vi "COMMAND_GetError.vi"(8 "error in (no error)":errorcluster, 11 "StageMH100301DMC in":refnum<class "StageMH100301DMC.lvclass">) -> (0 "error out":errorcluster, 3 "StageMH100301DMC out":refnum<class "StageMH100301DMC.lvclass">)   [LabVIEW 2010, in "StageMH100301DMC.lvclass"]
uses:
  StageMH100301DMC.lvclass
  StageMH100301DMC.lvclass/StageMH100301DMC.ctl
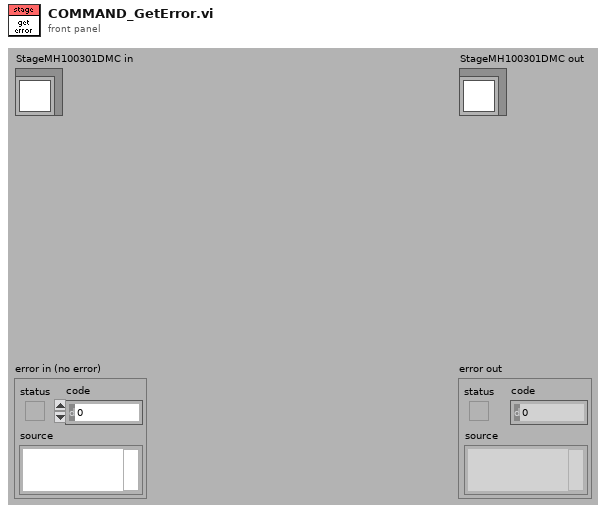
[diagram p1: front panel]
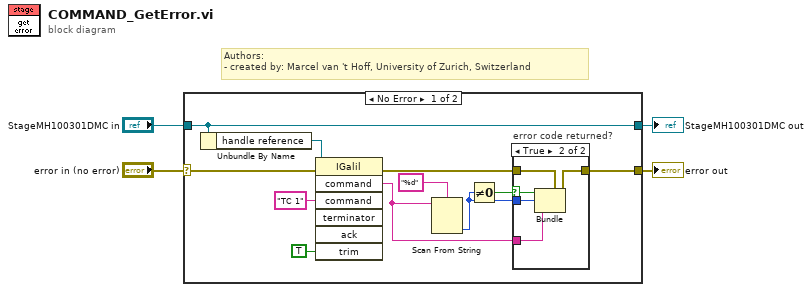
[diagram p0: block diagram]
diagram:
  # "Authors: \n- created by: Marcel van 't Hoff, University of Zurich, Switzerland"
  n1 = case shown="No Error" "error in (no error)" {
    selector: "error in (no error)" -> [w8 w23]
    tunnel: [w15 w23] -> w3
    tunnel: [w14 w22] -> w1
    tunnel: "StageMH100301DMC in" -> [w14 w22]
    frame No Error {
      n2 = Unbundle By Name(w14) -> ("handle reference"=w9:refnum<k7>)
      n3 = invoke class="IGalil" method="command"(reference=w9, error in=w8, "command"="TC 1", "trim"=TRUE) -> (error out=w5:errorcluster, "command"=w7:string)  [unwired: 3 in, 5 out]
      n4 = Scan From String(format string="%d", input string=w7) -> (output 1=w13:i32)  [unwired: 2 in, 4 out]
      n5 = Not Equal To 0?(x=w13) -> (x != 0?=w12:bool)
      n6 = case "error code returned?" shown="True" w12 {
        selector: w12 -> [_ w17]
        tunnel: w7 -> [_ w21]
        tunnel: w13 -> [_ w20]
        tunnel: w5 -> [w16 w19]
        tunnel: [w16 w18] -> w15
        frame False {
        }
        frame True {
          n7 = Bundle(cluster=w19, "status"=w17, "code"=w20, "source"=w21) -> (w18:errorcluster)
        }
      }
    }
    frame Error {
    }
  }
  "error out" <- w3
  "StageMH100301DMC out" <- w1
